vi "DaqNavi test.vi"() -> ()   [LabVIEW 2017]
uses:
  <userlib>/DAQNavi Polymorphic VI/create/DAQNavi Create Channel(AI-Voltage).vi
  <userlib>/DAQNavi Polymorphic VI/configure/timing/DAQNavi Timing(Convert Clock).vi
  <userlib>/DAQNavi Polymorphic VI/configure/DAQNavi Get Property/AI/DAQNaviGet_AI_ConvertClock_Rate.vi
  <userlib>/DAQNavi Polymorphic VI/configure/DAQNavi Get Property/AI/DAQNaviGet_AI_Trigger_Source.vi
  <userlib>/DAQNavi Polymorphic VI/read/DAQNavi Read (Analog 1D Wfm NChan NSamp).vi
panel:
  out "trigger source":string
  out "data 2":waveform(dbl)[](array[waveform])
  out "error out 4":errorcluster
  out "error out 3":errorcluster
  out "error out 2":errorcluster
  out "error out":errorcluster
  in  "samples per channel":u32=1000
  in  "rate":dbl=1000.0
  out "TASK USB 0":i32
  out "value range 0":string="+/- 5 V" caption="property value"
  out "physical channels 0":string="DemoDevice,BID#0/ai0:1" caption="property value"
  out "convert rate 0":dbl
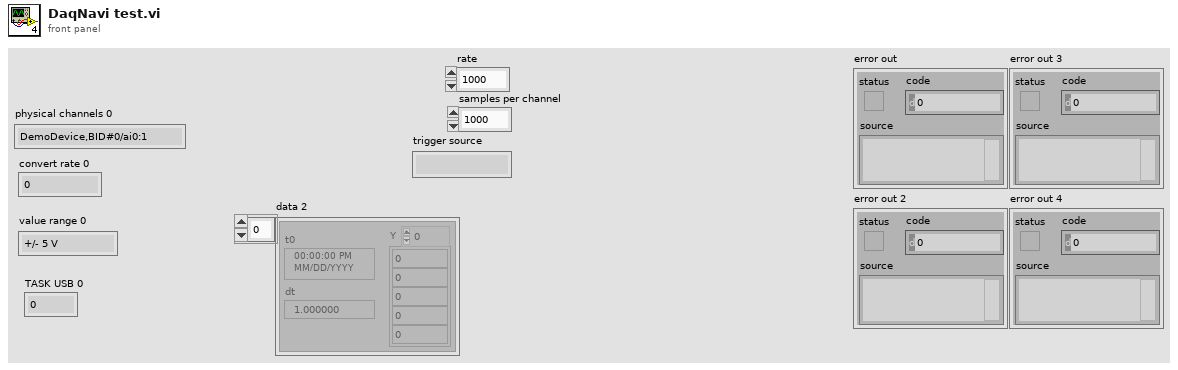
[diagram p1: front panel]
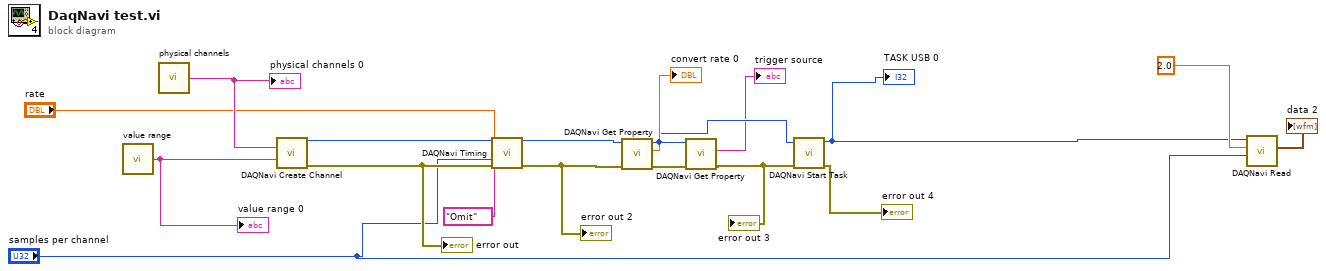
[diagram p0: block diagram]
diagram:
  n1 = call "value range"() -> ("property value"=w18:string)  [unwired: 1 out]
  "value range 0" <- w18
  n2 = call "physical channels"() -> ("property value"=w17:string)  [unwired: 1 out]
  "physical channels 0" <- w17
  n3 = call-poly <userlib>:"DAQNavi Create Channel.vi"("physical channels"=w17, "value range"=w18) -> ("task out"=w14:i32, "error out"=w12:errorcluster)  [unwired: 3 in, 9 out]
  "error out" <- w12
  n4 = call-poly <userlib>:"DAQNavi Timing.vi"("task in"=w14, "clock source"="Omit", "rate"="rate", "samples per channel"="samples per channel", "error in (no error)"=w12) -> ("task out"=w15:i32, "error out"=w11:errorcluster)  [unwired: 1 in, 8 out]
  "error out 2" <- w11
  n5 = call-poly <userlib>:"DAQNavi Get Property.vi"("error in (no error)"=w11, "task in"=w15) -> ("error out"=w2:errorcluster, "rate"=→"convert rate 0":dbl, "task out"=w5:i32)  [unwired: 7 out]
  n6 = call-poly <userlib>:"DAQNavi Get Property.vi"("error in (no error)"=w2, "task in"=w5) -> ("error out"=w3:errorcluster, "trigger source"=→"trigger source":string)  [unwired: 1 in, 7 out]
  "error out 3" <- w3
  n7 = call <userlib>:"DAQNavi Start Task.vi"("error in (no error)"=w3, "task in"=w5) -> ("error out"=→"error out 4":errorcluster, "task out"=w1:i32)  [unwired: 8 in]
  "TASK USB 0" <- w1
  n8 = call-poly <userlib>:"DAQNavi Read.vi"("number of samples per channel to read"="samples per channel", "timeout"=2.0, "task in"=w1) -> ("data"=→"data 2":waveform(dbl)[])  [unwired: 1 in, 7 out]
